vi "Begin FDMR plus measurement.vi"(9 "VID control":T4 {"Multip" items=["1"=1, "2"=2, "3"=3, "4"=4, "6"=6, "8"=8, "9"=9]; "AMC" items=["9"=9, "12"=12]}, 10 "FDMR+ script line":T2={"F_start [GHz]"=0.0, "F_end [GHz]"=0.0, "Field [T]"=0.0, "Points [-]"=0, "Sampling Rate"=15, "ModA [G]"=0.0, "ModF [kHz]"=0.0, "Time const [ms]"=0.0, "Angle [°]"=3.0, "Tmp [K]"=2.0, "Wait [min]"=0.0, "Repeat [-]"=1048576, "Comment"="", "Execute"=FALSE, "Auto-mod"=FALSE} {"Sampling Rate" items=["117 ks/S"=9, "58.6 kS/s"=10, "29.3 kS/s"=11, "14.6 kS/s"=12, "7.32 kS/s"=13, "3.66 kS/s"=14, "1.83 kS/s"=15]; "Time const [ms]" format="%_2e"; "ModF [kHz]" min=0.2 max=120.0; "Repeat [-]" max=1048576; "Tmp [K]" min=-1.0 max=330.0; "Field [T]" min=-16.0 max=16.0}, 11 "Referencies in":T1) -> (0 "error out":errorcluster)   [LabVIEW 2024]
uses:
  Datatypes/THz parameters.ctl
  Datatypes/FDMR+ script line.ctl
  Subsystem modules/Lock-in module/ctl/OSC sampling rate.ctl
  Subsystem modules/Messenger service/Data types/Messenger referencies.ctl
  Subsystem modules/Lock-in module/ctl/MFLI_message for module.ctl
  Subsystem modules/Lock-in module/ctl/MFLI_command enum.ctl
  Subsystem modules/THz module/ctl/THz Message for module.ctl
  Subsystem modules/THz module/ctl/THz commands enum.ctl
  Subsystem modules/THz module/ctl/THz sweep parameters.ctl
  Subsystem modules/Lock-in module/ctl/Mode.ctl
  Subsystem modules/Lock-in module/Lock-in module.lvlib
  Subsystem modules/THz module/THz source modeule.lvlib
  Subsystem modules/Messenger service/MessengerLib.lvlib
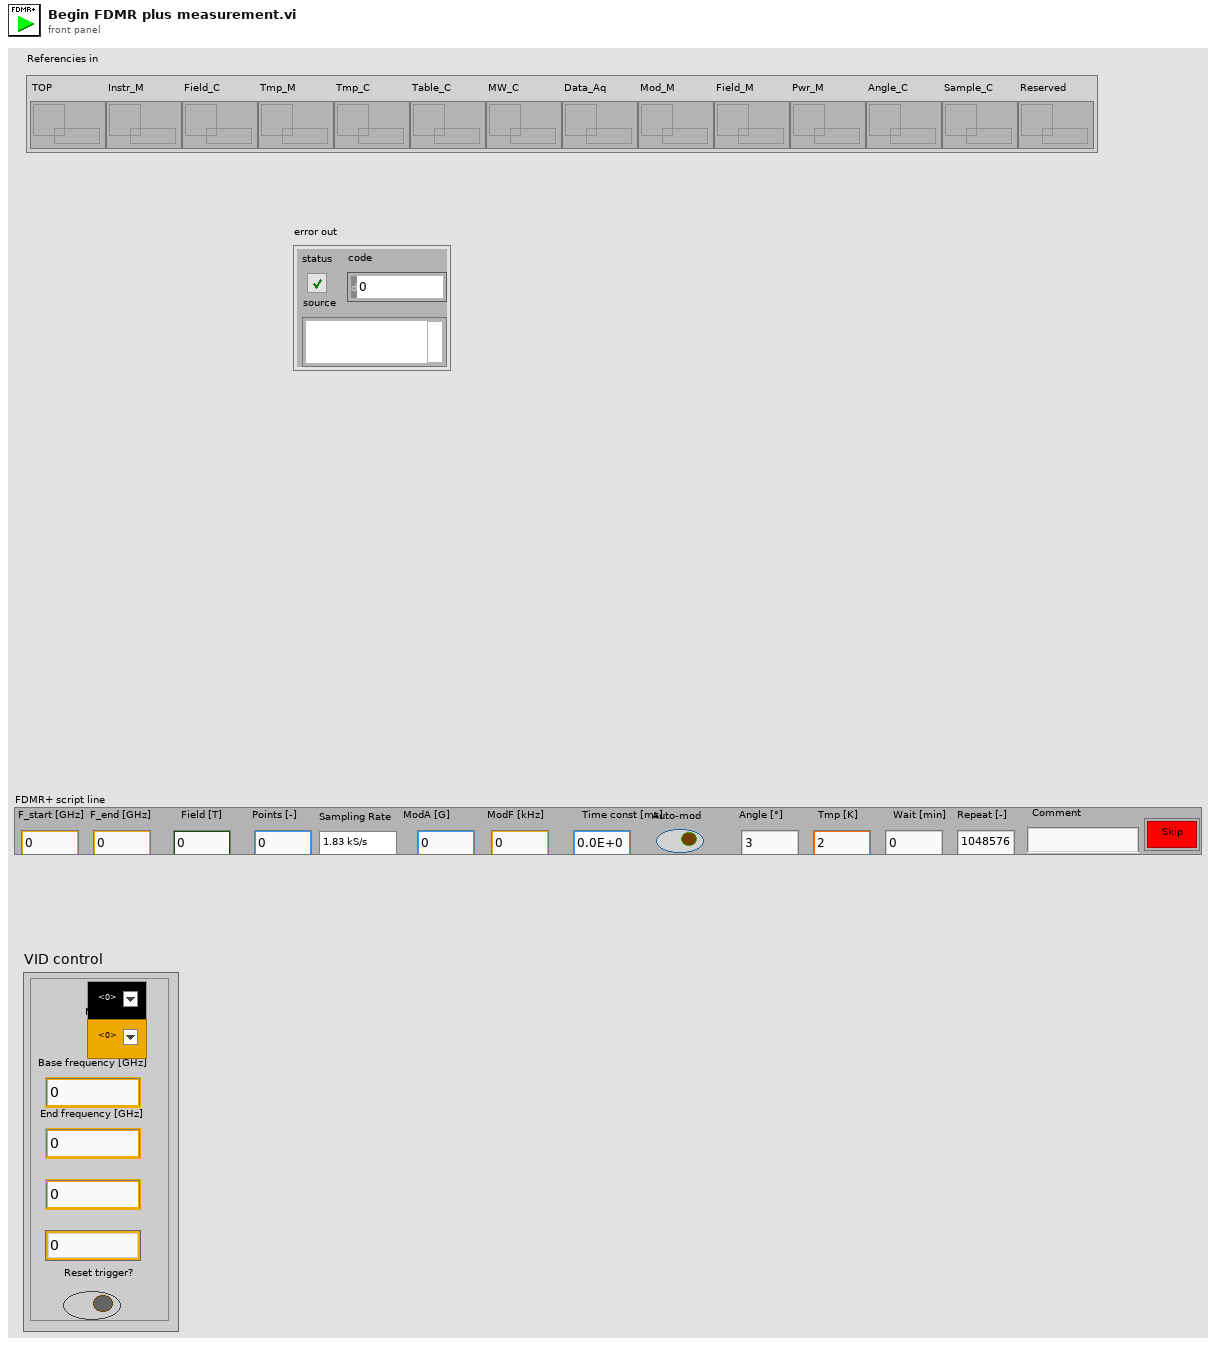
[diagram p1: front panel]
types:
  T1 = typedef "MessengerLib.lvlib/Messenger referencies.ctl" = cluster{"TOP":refnum<queue>, "Instr_M":refnum<queue>, "Field_C":refnum<queue>, "Tmp_M":refnum<queue>, "Tmp_C":refnum<queue>, "Table_C":refnum<queue>, "MW_C":refnum<queue>, "Data_Aq":refnum<queue>, "Mod_M":refnum<queue>, "Field_M":refnum<queue>, "Pwr_M":refnum<queue>, "Angle_C":refnum<queue>, "Sample_C":refnum<queue>, "Reserved":refnum<queue>}
  T2 = typedef "FDMR+ script line.ctl" = cluster{"F_start [GHz]":dbl, "F_end [GHz]":dbl, "Field [T]":dbl, "Points [-]":u32, "Sampling Rate":T3, "ModA [G]":dbl, "ModF [kHz]":dbl, "Time const [ms]":dbl, "Angle [°]":dbl, "Tmp [K]":dbl, "Wait [min]":dbl, "Repeat [-]":i32, "Comment":string, "Execute":bool, "Auto-mod":bool}
  T3 = typedef "OSC sampling rate.ctl" = u16
  T4 = typedef "THz parameters.ctl" = cluster{"AMC":u16, "Multip":u16, "Base frequency [GHz]":dbl, "End frequency [GHz]":dbl, "Im frequency [MHz]":dbl, "Sweep up [ms]":dbl, "Reset trigger?":bool}
  T5 = typedef "Lock-in module.lvlib/Mode.ctl" = enum16{"None", "Point", "Scope", "Both", "DAQ"}
  T6 = typedef "THz source modeule.lvlib/THz sweep parameters.ctl" = cluster{"Start [GHz]":dbl, "End [GHz] ":dbl, "Sweep up\ntime [ms]":dbl, "Sweep down\ntime [ms]":dbl, "Intermidiate [MHz]":dbl, "Reset trigger":bool}
  T7 = typedef "THz source modeule.lvlib/THz Message for module.ctl" = cluster{"Command":T8, "Data":variant}
  T8 = typedef "THz source modeule.lvlib/THz commands enum.ctl" = enum16{"Ignore", "Connect", "Update", "Set parameters", "Disconnect", "End"}
  T9 = typedef "Lock-in module.lvlib/MFLI_message for module.ctl" = cluster{"Command":T10, "Data":variant}
  T10 = typedef "Lock-in module.lvlib/MFLI_command enum.ctl" = enum16{"Initialize", "Update", "Set parameters", "Set module", "Set individual parameters", "Get point", "Get array", "Disconnect", "End", "Ignore"}
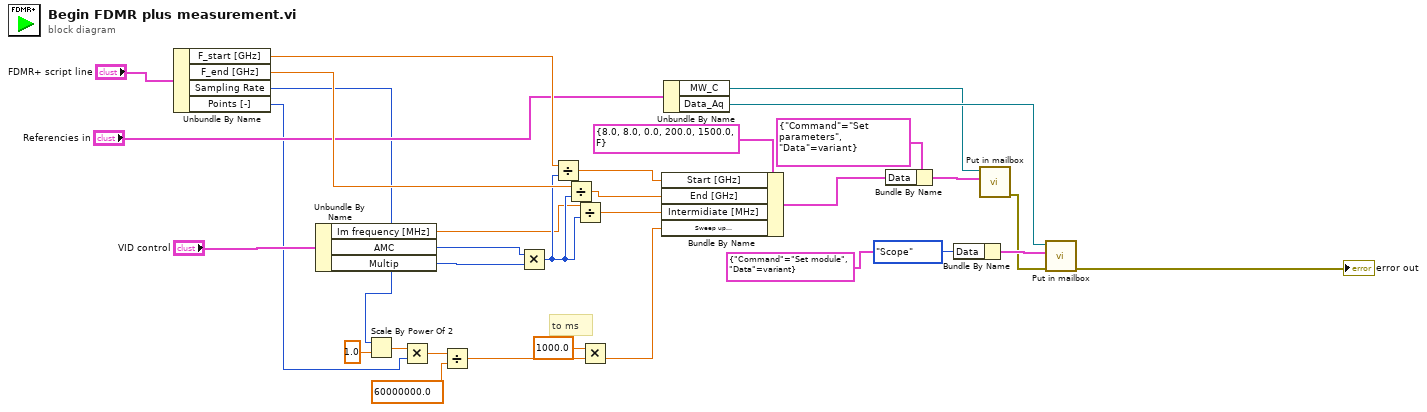
[diagram p0: block diagram]
diagram:
  # "to ms"
  n1 = Unbundle By Name("FDMR+ script line") -> ("F_start [GHz]"=w31:dbl, "F_end [GHz]"=w32:dbl, "Sampling Rate"=w10:T3, "Points [-]"=w7:u32)
  n2 = Unbundle By Name("VID control") -> ("Im frequency [MHz]"=w1:dbl, "AMC"=w18:u16, "Multip"=w19:u16)
  n3 = Scale By Power Of 2(n=w10, x=1.0 ("y")) -> (x*2^n=w8:dbl)
  n4 = Multiply(x=w8, y=w7) -> (x*y=w6:dbl)
  n5 = Divide(x=w6, y=60000000.0) -> (x/y=w4:dbl)
  n6 = Multiply(x=w18, y=w19) -> (x*y=w20:u16)
  n7 = Divide(x=w31, y=w20) -> (x/y=w13:dbl)
  n8 = Divide(x=w32, y=w20) -> (x/y=w14:dbl)
  n9 = Divide(x=w1, y=w20) -> (x/y=w17:dbl)
  n10 = Multiply(x=1000.0, y=w4) -> (x*y=w3:dbl)
  n11 = Bundle By Name(cluster=T6 {"Start [GHz]"=8.0, "End [GHz] "=8.0, "Sweep up\ntime [ms]"=0.0, "Sweep down\ntime [ms]"=200.0, "Intermidiate [MHz]"=1500.0, "Reset trigger"=FALSE} ("Sweep parameters"), "Start [GHz]"=w13, "End [GHz]"=w14, "Intermidiate [MHz]"=w17, "Sweep up\ntime [ms]"=w3) -> (w15:T6)
  n12 = Unbundle By Name("Referencies in") -> ("MW_C"=w12:refnum<queue>, "Data_Aq"=w27:refnum<queue>)
  n13 = Bundle By Name(cluster=T7 {"Command"=enum."Set parameters", "Data"=variant} ("Incoming msg"), "Data"=w15) -> (w16:T7)
  n14 = Bundle By Name(cluster=T9 {"Command"=enum."Set module", "Data"=variant} ("MSG for  ACQ"), "Data"=Mode."Scope" ("Mode")) -> (w29:T9)
  n15 = call "Put in mailbox.vi"("Message"=w16, "Queue in"=w12) -> ("error out"=w28:errorcluster)  [unwired: 7 in, 2 out]
  n16 = call "Put in mailbox.vi"("error in (no error)"=w28, "Message"=w29, "Queue in"=w27) -> ("error out"=→"error out":errorcluster)  [unwired: 6 in, 2 out]
